vi "Select Item.vi"(8 "error in (no error)":errorcluster, 9 "Update internal index":bool, 10 "Item index":i32, 11 "Batch Processor in":refnum<class "Batch Processor.lvclass">) -> (0 "error out":errorcluster, 3 "Batch Processor out":refnum<class "Batch Processor.lvclass">)   [LabVIEW 2020, in "Batch Processor.lvclass"]
uses:
  Batch Processor.lvclass
  Batch Processor.lvclass/Batch Processor.ctl
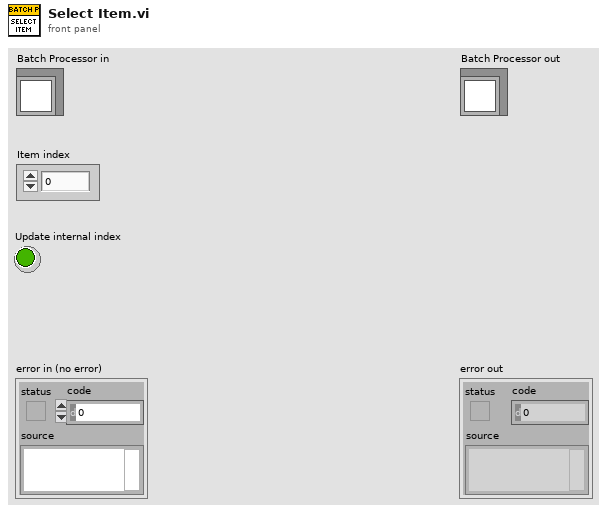
[diagram p1: front panel]
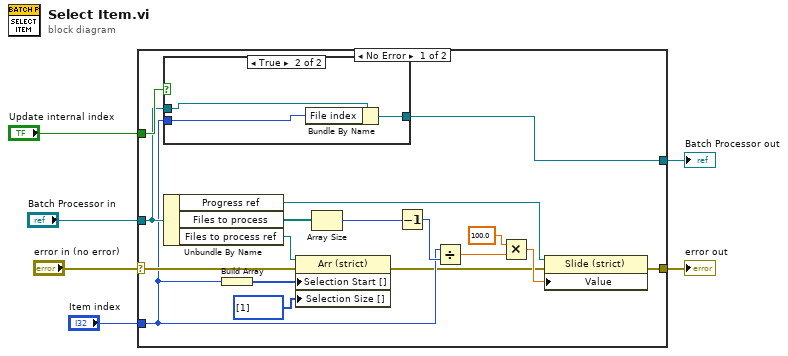
[diagram p0: block diagram]
diagram:
  n1 = case shown="No Error" "error in (no error)" {
    selector: "error in (no error)" -> [w20 w29]
    tunnel: [w7 w29] -> w5
    tunnel: [w17 w28] -> w3
    tunnel: "Batch Processor in" -> [w18 w28]
    tunnel: "Item index" -> [w13 _]
    tunnel: "Update internal index" -> [w19 _]
    frame No Error {
      n2 = case shown="True" w19 {
        tunnel: w18 -> [w24 w27]
        tunnel: [w24 w26] -> w17
        tunnel: w13 -> [_ w25]
        frame False {
        }
        frame True {
          n3 = Bundle By Name(cluster=w27, "File index"=w25) -> (w26:refnum<class "Batch Processor.lvclass">)
        }
      }
      n4 = Unbundle By Name(w18) -> ("Progress ref"=w10:refnum<vi>, "Files to process"=w16:path[], "Files to process ref"=w23:refnum<vi>)
      n5 = Build Array(w13) -> (w22:i32[])
      n6 = property class="Arr (strict)"(reference=w23, error in=w20, "Selection Start []"=w22, "Selection Size []"=i32[] [1]) -> (error out=w8:errorcluster)  [unwired: 1 out]
      n7 = Array Size(array=w16) -> (size(s)=w15:i32)
      n8 = Decrement(x=w15) -> (x-1=w14:i32)
      n9 = Divide(x=w13, y=w14) -> (x/y=w12:dbl)
      n10 = Multiply(x=100.0, y=w12) -> (x*y=w9:dbl)
      n11 = property class="Slide (strict)"(reference=w10, error in=w8, "Value"=w9) -> (error out=w7:errorcluster)  [unwired: 1 out]
    }
    frame Error {
    }
  }
  "error out" <- w5
  "Batch Processor out" <- w3
